vi "Listbox Properties.vi"(8 "error in (no error)":errorcluster, 11 "Configuration File Variable List 2":refnum<vi>) -> (0 "error out":errorcluster)   [LabVIEW 2013]
doc: "This vi sets the properties for multicolumn listbox\n[input]\nConfiguration reference\nError in\n[output]\nError out"
panel:
  in  "Configuration File Variable List":i32[](listbox)
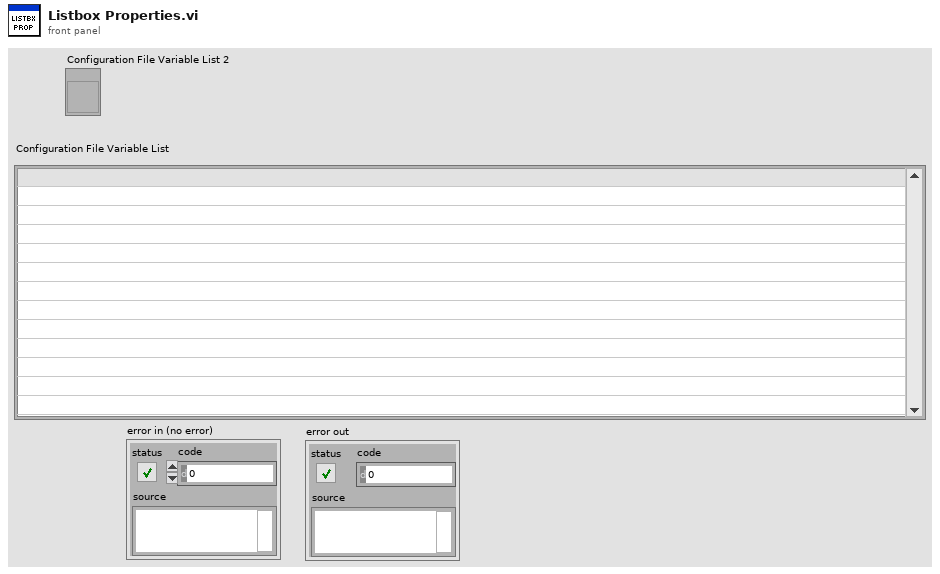
[diagram p1: front panel]
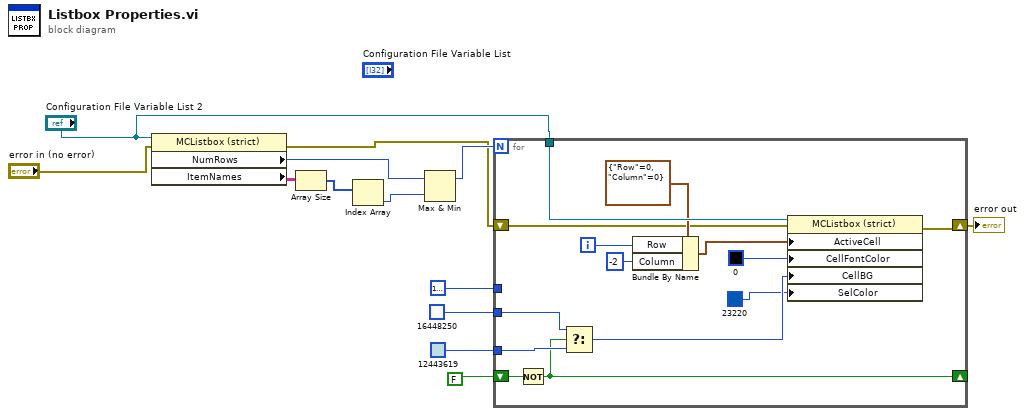
[diagram p0: block diagram]
diagram:
  n1 = property class="MCListbox (strict)"(reference="Configuration File Variable List 2", error in="error in (no error)") -> (error out=w4:errorcluster, "NumRows"=w10:u32, "ItemNames"=w13:string[][])  [unwired: 1 out]
  n2 = Array Size(array=w13) -> (size(s)=w12:i32[])
  n3 = Index Array(array=w12) -> (element=w11:i32)  [unwired: 1 in]
  n4 = Max & Min(x=w10, y=w11) -> (max(x,y)=w9:u32)  [unwired: 1 out]
  n5 = for {
    N: w9 -> [_]
    tunnel: "Configuration File Variable List 2" -> [w27]
    tunnel: u32 16448250 ("Color") -> [w19]
    tunnel: u32 12443619 ("Color") -> [w23]
    shift-right: [w21] -> _
    shift-left: FALSE -> [w22]
    tunnel: u32 16777226 ("Color") -> [_]
    shift-right: [w17] -> w1
    shift-left: w4 -> [w18]
    i -> [w25]
    n6 = Not(x=w22) -> (.not. x?=w21:bool)
    n7 = Select(t=w19, s=w21, f=w23) -> (s? t:f=w20:u32)
    n8 = Bundle By Name(cluster=cluster{"Row":i32, "Column":i32} {"Row"=0, "Column"=0}, "Row"=w25, "Column"=-2) -> (w16:cluster{"Row":i32, "Column":i32})
    n9 = property class="MCListbox (strict)"(reference=w27, error in=w18, "ActiveCell"=w16, "CellFontColor"=u32 0 ("Color"), "CellBG"=w20, "SelColor"=u32 23220 ("Color")) -> (error out=w17:errorcluster)  [unwired: 1 out]
  }
  "error out" <- w1
